vi "setBeginDirectOrKickoff.vi"(8 "error in (no error)":errorcluster, 10 "Game in":refnum<class "Game.lvclass">, 11 "Play in":refnum<class "Play.lvclass">) -> (0 "error out":errorcluster, 2 "Game out":refnum<class "Game.lvclass">, 3 "Play out":refnum<class "Play.lvclass">)   [LabVIEW 2023, in "Play.lvclass"]
uses:
  Play.lvclass
  Game_class/Game.lvclass
  Game_class/Game.lvclass/Game.ctl
  Ally_class/Ally.lvclass/Ally.ctl
  Game_class/Read OffensiveTeam.vi
  Ally_class/Write DirectOrKickoff.vi
  Game_class/Write OffensiveTeam.vi
  Ally_class/Ally.lvclass
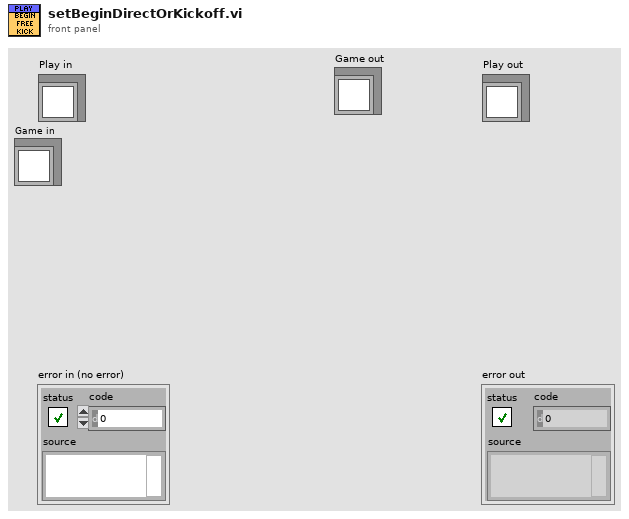
[diagram p1: front panel]
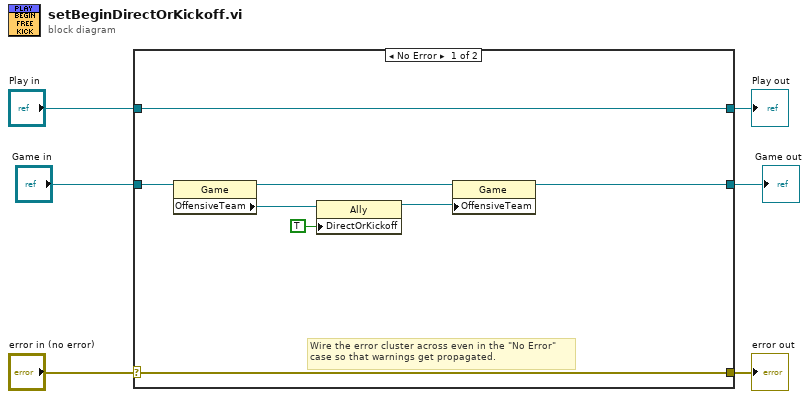
[diagram p0: block diagram]
diagram:
  n1 = case shown="No Error" "error in (no error)" {
    selector: "error in (no error)" -> [w13 w16]
    tunnel: [w13 w16] -> w5
    tunnel: [w14 w15] -> w3
    tunnel: "Play in" -> [w14 w15]
    tunnel: "Game in" -> [w12 _]
    tunnel: [w7 _] -> w1
    frame No Error {
      # "Wire the error cluster across even in the \"No Error\"\ncase so that warnings get propagated."
      n2 = property class="Game"(reference=w12) -> (reference out=w9:refnum<class "Game.lvclass">, "OffensiveTeam"=w11:refnum<class "Ally.lvclass">)  [unwired: 1 in, 1 out]
      n3 = property class="Ally"(reference=w11, "DirectOrKickoff"=TRUE) -> (reference out=w8:refnum<class "Ally.lvclass">)  [unwired: 1 in, 1 out]
      n4 = property class="Game"(reference=w9, "OffensiveTeam"=w8) -> (reference out=w7:refnum<class "Game.lvclass">)  [unwired: 1 in, 1 out]
    }
    frame Error {
    }
  }
  "error out" <- w5
  "Play out" <- w3
  "Game out" <- w1
